vi "Is a Dqmh Event.vi"(8 "error in":errorcluster, 11 "VI Refnum":refnum<vi>) -> (0 "error out":errorcluster, 2 "Event Type":T1=enum."Request", 3 "Is Dqmh Event":bool)   [LabVIEW 2021, in "TAF Proj Document Type.lvlib" / "Project Parser.lvlib"]
uses:
  <vilib>/Wovalab/AntiDoc/Document Type/Add-ons/LabVIEW TAF Project/Project Parser/Project Parser.lvlib
  <vilib>/Wovalab/AntiDoc/Document Type/Add-ons/LabVIEW TAF Project/Project Parser/Dqmh Event Type--enum.ctl
  <vilib>/UserTags/UserTags.lvlib
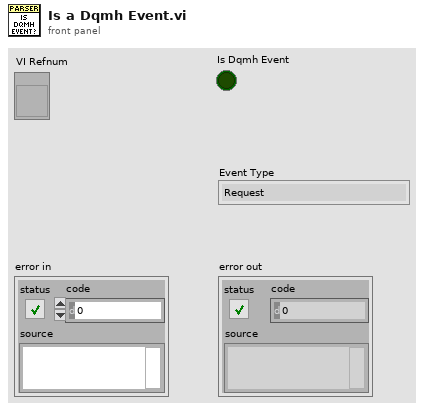
[diagram p1: front panel]
types:
  T1 = typedef "TAF Proj Document Type.lvlib/Project Parser.lvlib/Dqmh Event Type--enum.ctl" = enum16{"Not a DQMH Event", "Request", "Request And Wait For Reply", "Broadcast"}
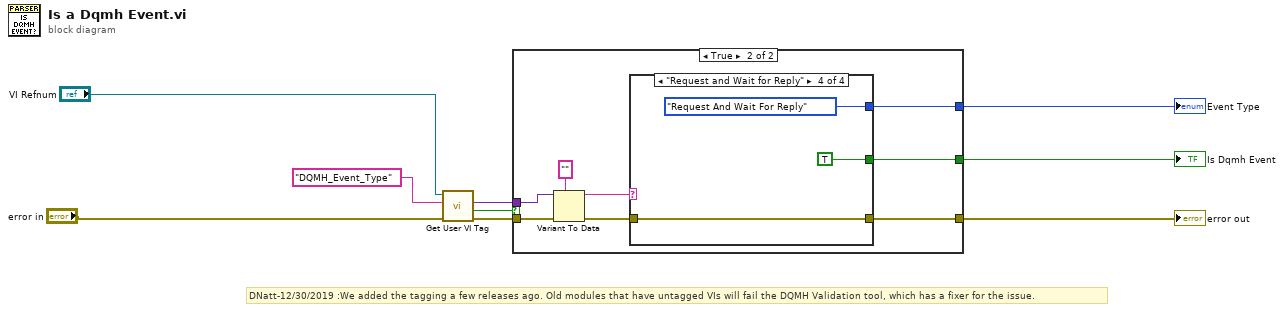
[diagram p0: block diagram]
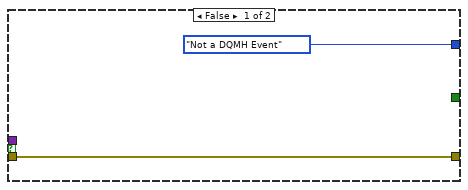
[diagram p2: hidden frame]
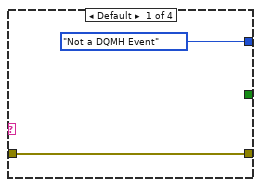
[diagram p3: hidden frame]
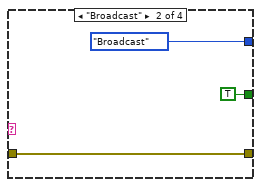
[diagram p4: hidden frame]
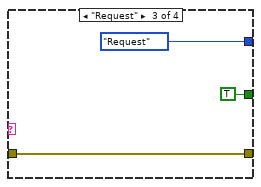
[diagram p5: hidden frame]
diagram:
  # "DNatt-12/30/2019 :We added the tagging a few releases ago. Old modules that have untagged VIs will fail the DQMH Validation tool, which has a fixer for the issue."
  n1 = call <vilib>:"Get User VI Tag.vi"("error in (no error)"="error in", "Tag Name"="DQMH_Event_Type", "VI Refnum"="VI Refnum") -> ("error out"=w3:errorcluster, "Was Tag Found?"=w2:bool, "Value"=w1:variant)  [unwired: 5 in, 1 out]
  n2 = case shown="True" w2 {
    tunnel: w3 -> [w10 w19]
    tunnel: w1 -> [_ w18]
    tunnel: [Dqmh_Event_Type--enum."Not a DQMH Event" ("Event Type") w13] -> w6
    tunnel: [w10 w15] -> w8
    tunnel: [_ w12] -> w5
    frame False {
    }
    frame True {
      n3 = Variant To Data(error in=w19, type="", Variant=w18) -> (data=w16:string, error out=w14:errorcluster)
      n4 = case shown="\"Request and Wait for Reply\"" w16 {
        tunnel: [w21 w23 w26 w29] -> w15
        tunnel: w14 -> [w21 w23 w26 w29]
        tunnel: [Dqmh_Event_Type--enum."Not a DQMH Event" ("Event Type") Dqmh_Event_Type--enum."Broadcast" ("Event Type") Dqmh_Event_Type--enum."Request" ("Event Type") Dqmh_Event_Type--enum."Request And Wait For Reply" ("Event Type")] -> w13
        tunnel: [_ TRUE TRUE TRUE] -> w12
        frame Default {
        }
        frame "Broadcast" {
        }
        frame "Request" {
        }
        frame "Request and Wait for Reply" {
        }
      }
    }
  }
  "error out" <- w8
  "Is Dqmh Event" <- w5
  "Event Type" <- w6
